vi "Global - UI Stream and Variable Connections.vi"() -> ()   [LabVIEW 2013]
uses:
  support/Message Queue/Message Cluster.ctl
  controls/Variable References.ctl
  controls/Raw Values.ctl
  controls/FPGA State.ctl
  controls/Controller Calcs.ctl
  controls/Observer Calcs.ctl
  controls/Other Calcs.ctl
  support/Message Queue/Message Queue.lvlib
panel:
  in  "Variable References":T1
  in  "RT Message Stream":refnum<k21>
  in  "UI Command Stream":refnum<k21>
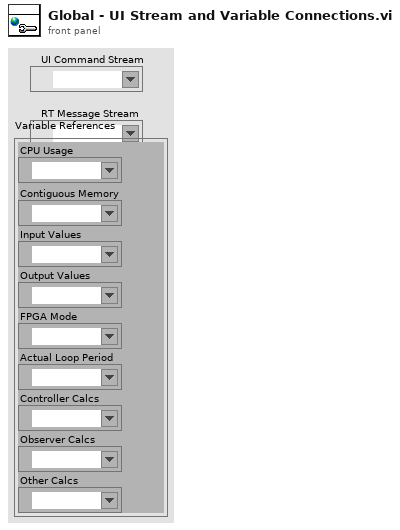
[diagram p1: front panel]
types:
  T1 = typedef "Variable References.ctl" = cluster{"CPU Usage":refnum<k21>, "Contiguous Memory":refnum<k21>, "Input Values":refnum<k21>, "Output Values":refnum<k21>, "FPGA Mode":refnum<k21>, "Actual Loop Period":refnum<k21>, "Controller Calcs":refnum<k21>, "Observer Calcs":refnum<k21>, "Other Calcs":refnum<k21>}
diagram:
